vi "Fibonacci.vi"() -> ()   [LabVIEW 2015]
panel:
  out "Output":i32[](array[numeric])
  in  "Input_num":i32=1
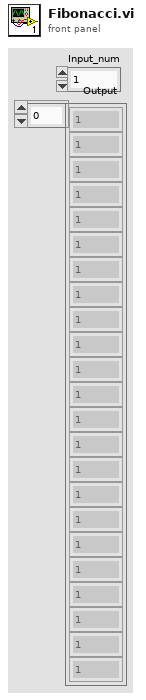
[diagram p1: front panel]
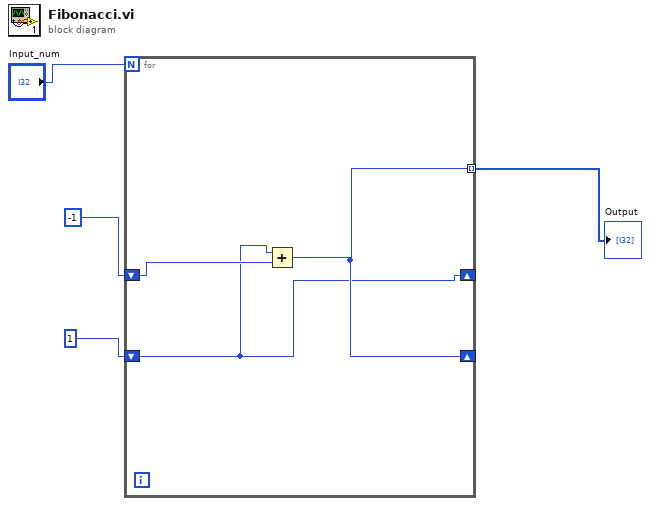
[diagram p0: block diagram]
diagram:
  n1 = for {
    N: "Input_num" -> [_]
    shift-right: [w5] -> _
    shift-left: -1 -> [w7]
    shift-right: [w6] -> _
    shift-left: 1 -> [w5]
    tunnel: [w6] -> w1 mode=indexing
    n2 = Add(x=w5, y=w7) -> (x+y=w6:i32)
  }
  "Output" <- w1
